vi "SetByteOrder.vi"(8 "Error In":errorcluster, 10 "Byte Order":T1, 11 "Keithley 6482 In":refnum<visa-resource-name>) -> (0 "Error Out":errorcluster, 3 "Keithley 6482 Out":refnum<visa-resource-name>)   [LabVIEW 2012, in "Keithley-6482.lvlib"]
uses:
  Keithley-6482.lvlib
  Controls/ByteOrder.ctl
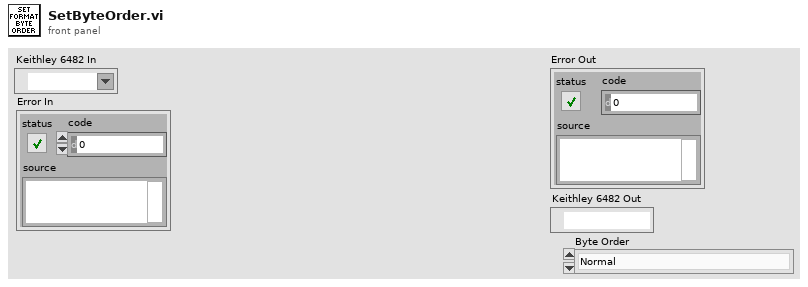
[diagram p1: front panel]
types:
  T1 = typedef "Keithley-6482.lvlib/ByteOrder.ctl" = enum16{"Normal", "Swapped"}
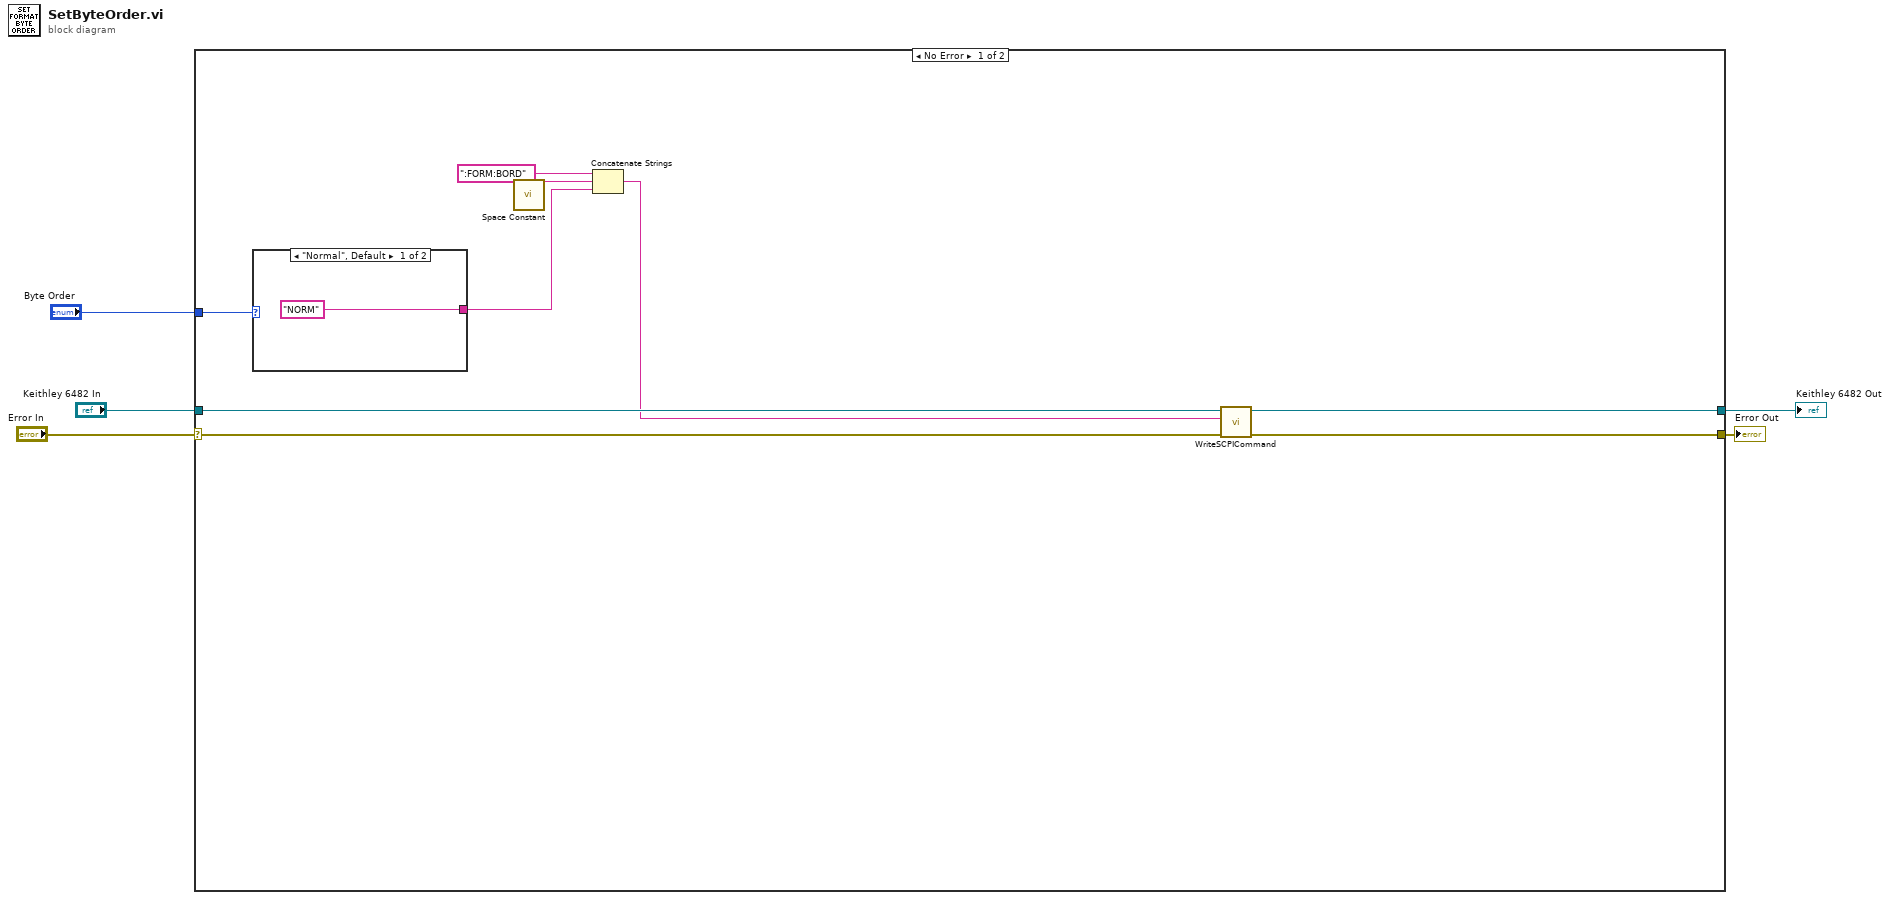
[diagram p0: block diagram]
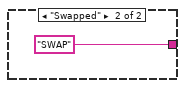
[diagram p2: hidden frame]
diagram:
  n1 = case shown="No Error" "Error In" {
    selector: "Error In" -> [w8 w17]
    tunnel: "Keithley 6482 In" -> [w7 w18]
    tunnel: [w9 w17] -> w3
    tunnel: [w10 w18] -> w2
    tunnel: "Byte Order" -> [w12 _]
    frame No Error {
      n2 = case shown="\"Normal\", Default" w12 {
        tunnel: ["NORM" "SWAP"] -> w11
        frame "Normal", Default {
        }
        frame "Swapped" {
        }
      }
      n3 = call <vilib>:"Space Constant.vi"() -> ("String"=w13:string)
      n4 = Concatenate Strings(":FORM:BORD", w13, w11) -> (w6:string)
      n5 = call "WriteSCPICommand.vi"("Error In"=w8, "SCPI Command"=w6, "Keithley 6482 In"=w7) -> ("Error Out"=w9:errorcluster, "Keithley 6482 Out"=w10:refnum<visa-resource-name>)  [unwired: 7 in]
    }
    frame Error {
    }
  }
  "Error Out" <- w3
  "Keithley 6482 Out" <- w2
